vi "SafetyStatus.vi"(0 "Universal Robot.lvclass in":refnum<class "Universal Robot.lvclass">, 5 "error in (no error)":errorcluster) -> (11 "safetyStatus out":T1, 14 "Universal Robot.lvclass out":refnum<class "Universal Robot.lvclass">, 19 "error out":errorcluster)   [LabVIEW 2019, in "Universal Robot.lvclass"]
uses:
  Universal Robot.lvclass
  SafetyStatus.ctl
  Universal Robot.lvclass/Universal Robot.ctl
  Client Interfaces/Dashboard Server/Dashboard Server.lvclass
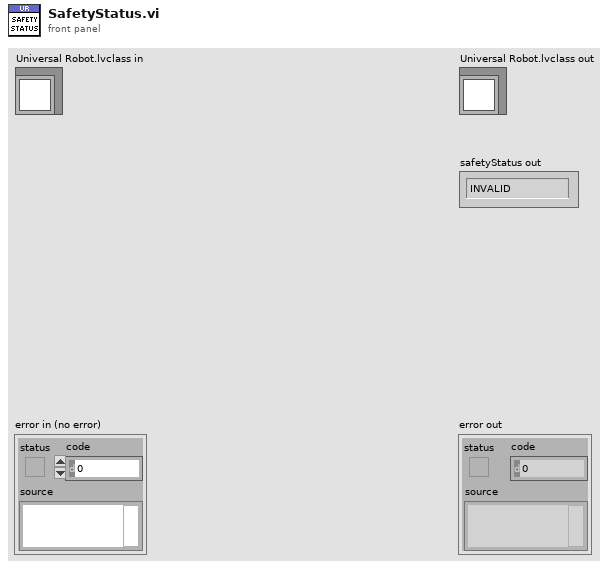
[diagram p1: front panel]
types:
  T1 = typedef "Universal Robot.lvclass/SafetyStatus.ctl" = enum16{"INVALID", "NORMAL", "REDUCED", "PROTECTIVE_STOP", "RECOVERY", "SAFEGUARD_STOP", "SYSTEM_EMERGENCY_STOP", "ROBOT_EMERGENCY_STOP", "VIOLATION", "FAULT", "AUTOMATIC_MODE_SAFEGAURD_STOP", "SYSTEM_THREE_POSITION_ENABLING_STOP"}
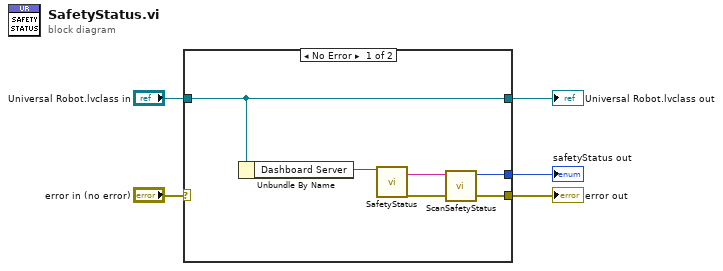
[diagram p0: block diagram]
diagram:
  n1 = case shown="No Error" "error in (no error)" {
    selector: "error in (no error)" -> [_ w12]
    tunnel: [w9 w12] -> w4
    tunnel: "Universal Robot.lvclass in" -> [w10 w11]
    tunnel: [w10 w11] -> w2
    tunnel: [w6 _] -> w1
    frame No Error {
      n2 = Unbundle By Name(w10) -> ("Dashboard Server"=w7:refnum<class "Dashboard Server.lvclass">)
      n3 = call-dynamic "SafetyStatus.vi"("DashboardServer in"=w7) -> ("safetyStatus"=w8:string, "error out"=w9:errorcluster)  [unwired: 16 in, 1 out]
      n4 = call "ScanSafetyStatus.vi"("safetyStatus in"=w8) -> ("safetyStatus out"=w6:T1)  [unwired: 10 in]
    }
    frame Error {
    }
  }
  "error out" <- w4
  "Universal Robot.lvclass out" <- w2
  "safetyStatus out" <- w1
